vi "Sincronizaciones.vi"() -> ()   [LabVIEW 2019]
panel:
  out "millisecond timer value INICIO":u32
  out "millisecond timer value":u32
  in  "Stop":bool
  out "Time Elapsed":u32
  out "Iteration":i32
  in  "Initialize?":bool
  # "When you pre-initialize, the time-elapsed inditcator\nshould read 5000 when the iteration is non-zero. The first\niteration \"0\" will still be off because of the initial timestamp\nfrom outside the loop, but the first actual iteration is in fact\nstill taking 5 seconds.\n\nWithout pre-initializing, the actual loop time will be some value\nbetween 0 and the constant 5000 on the first iteration."
  # "Note: This VI will take\nup to 10 seconds to stop\nonce the button is pressed."
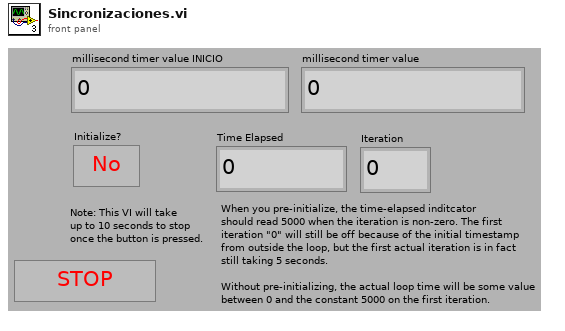
[diagram p1: front panel]
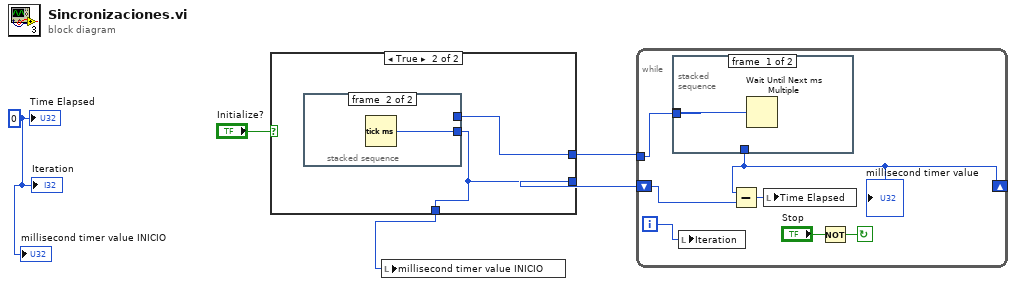
[diagram p0: block diagram]
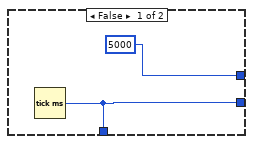
[diagram p2: hidden frame]
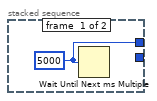
[diagram p3: hidden frame]
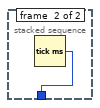
[diagram p4: hidden frame]
diagram:
  w3 = u32 0 ("Time Elapsed")
  n1 = case shown="True" "Initialize?" {
    tunnel: [w6 w8] -> w4
    tunnel: [5000 w9] -> w1
    tunnel: [w6 w8] -> w2
    frame False {
      n2 = Tick Count (ms)() -> (millisecond timer value=w6:u32)
    }
    frame True {
      n3 = stacked-sequence {
        tunnel: [_ w11] -> w8
        tunnel: [w10 _] -> w9
        frame #0 {
          w10 = u32 5000 ("millisecond multiple")
          n4 = Wait Until Next ms Multiple(millisecond multiple=w10) -> ()  [unwired: 1 out]
        }
        frame #1 {
          n5 = Tick Count (ms)() -> (millisecond timer value=w11:u32)
        }
      }
    }
  }
  n6 = local write "millisecond timer value INICIO"(w2) -> ()
  n7 = while {
    shift-right: [w17] -> _
    shift-left: w4 -> [w18]
    tunnel: w1 -> [w16]
    i -> [w12]
    stop <- w15 continue-if-true
    n8 = stacked-sequence {
      tunnel: [_ w20] -> w17
      tunnel: [w19 _] -> _
      tunnel: w16 -> [w19 _]
      frame #0 {
        n9 = Wait Until Next ms Multiple(millisecond multiple=w19) -> ()  [unwired: 1 out]
      }
      frame #1 {
        n10 = Tick Count (ms)() -> (millisecond timer value=w20:u32)
      }
    }
    "millisecond timer value" <- w17
    n11 = local write "Iteration"(w12) -> ()
    n12 = Subtract(x=w17, y=w18) -> (x-y=w13:u32)
    n13 = local write "Time Elapsed"(w13) -> ()
    n14 = Not(x="Stop") -> (.not. x?=w15:bool)
  }
  "Time Elapsed" <- w3
  "millisecond timer value INICIO" <- w3
  "Iteration" <- w3
